vi "Construct Data Block.vi"(8 "error in (no error)":errorcluster, 11 "Modbus Data Store in":refnum<class "MB Data Block.lvclass">) -> (0 "error out":errorcluster, 3 "Modbus Data Store out":refnum<class "MB Data Block.lvclass">)   [LabVIEW 2018, in "MB PLC Client.lvlib" / "MB Data Block.lvclass"]
uses:
  MB Data Block.lvclass
  MB Data Block.lvclass/MB Data Block.ctl
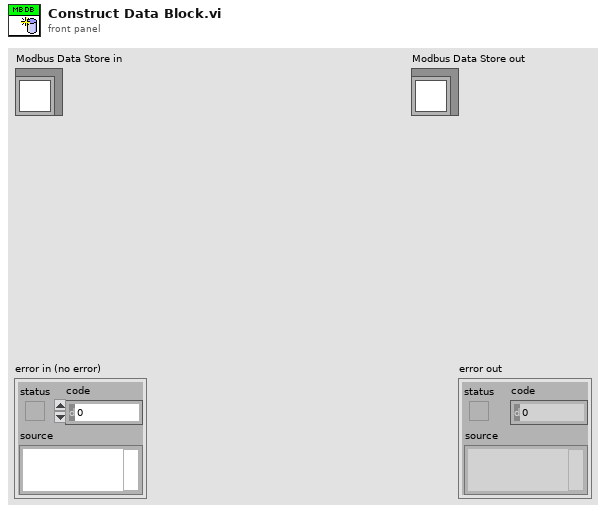
[diagram p1: front panel]
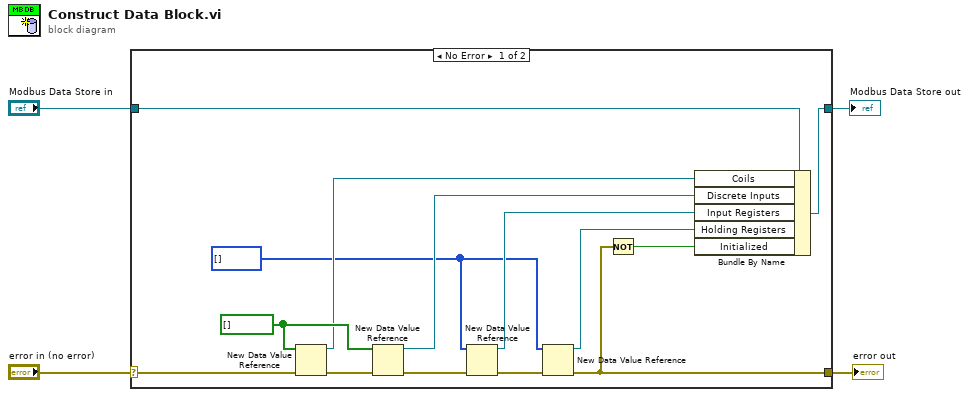
[diagram p0: block diagram]
diagram:
  n1 = case shown="No Error" "error in (no error)" {
    selector: "error in (no error)" -> [w18 w20]
    tunnel: [w6 w20] -> w3
    tunnel: "Modbus Data Store in" -> [w17 w19]
    tunnel: [w16 w19] -> w1
    frame No Error {
      w8 = u16[] []
      w14 = bool[] [] ("Coils")
      n2 = New Data Value Reference(data value=w14, error in=w18) -> (data value reference=w12:refnum<data-value>, error out=w15:errorcluster)
      n3 = New Data Value Reference(data value=w14, error in=w15) -> (data value reference=w13:refnum<data-value>, error out=w11:errorcluster)
      n4 = New Data Value Reference(data value=w8, error in=w11) -> (data value reference=w10:refnum<data-value>, error out=w9:errorcluster)
      n5 = New Data Value Reference(data value=w8, error in=w9) -> (data value reference=w7:refnum<data-value>, error out=w6:errorcluster)
      n6 = Not(x=w6) -> (.not. x?=w5:bool)
      n7 = Bundle By Name(cluster=w17, "Coils"=w12, "Discrete Inputs"=w13, "Input Registers"=w10, "Holding Registers"=w7, "Initialized"=w5) -> (w16:refnum<class "MB Data Block.lvclass">)
    }
    frame Error {
    }
  }
  "error out" <- w3
  "Modbus Data Store out" <- w1
